vi "SetParam.vi"(8 "error in (no error)":errorcluster caption="entrée d'erreur (pas d'erreur)", 10 "zero_one_loss":cluster{"normalize":bool, "sample_weight":dbl[]}={"normalize"=TRUE, "sample_weight"=[]}, 11 "Zero_One_Loss.lvclass":refnum<class "Zero_One_Loss.lvclass">) -> (0 "error out":errorcluster caption="sortie d'erreur", 3 "Zero_One_Loss.lvclass":refnum<class "Zero_One_Loss.lvclass">)   [LabVIEW 2020, in "Zero_One_Loss.lvclass"]
doc: "Set Parameters"
uses:
  Zero_One_Loss.lvclass
  Zero_One_Loss.lvclass/Zero_One_Loss.ctl
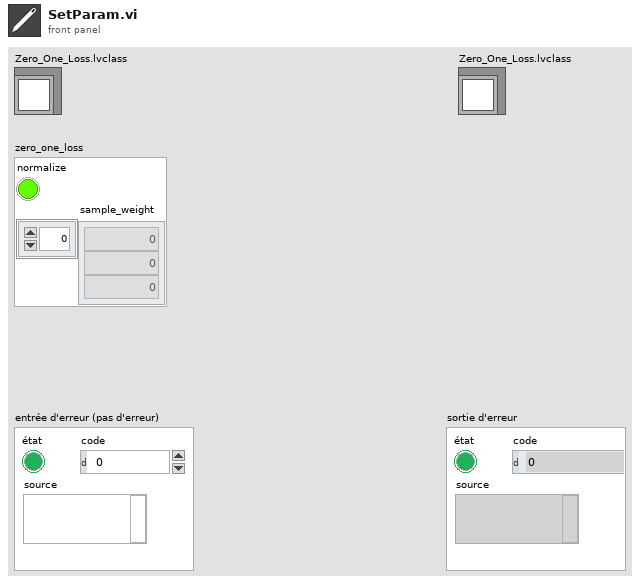
[diagram p1: front panel]
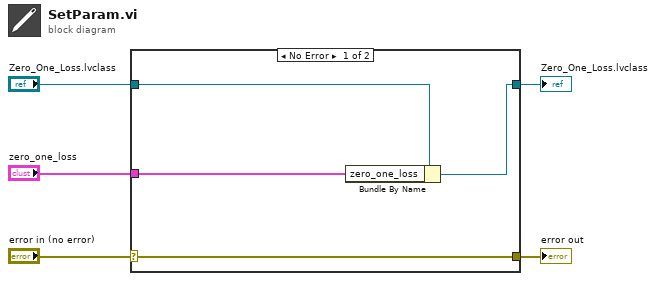
[diagram p0: block diagram]
diagram:
  n1 = case shown="No Error" "error in (no error)" {
    selector: "error in (no error)" -> [w9 w10]
    tunnel: [w9 w10] -> w4
    tunnel: [w7 w11] -> w2
    tunnel: "Zero_One_Loss.lvclass" -> [w8 w11]
    tunnel: "zero_one_loss" -> [w6 _]
    frame No Error {
      n2 = Bundle By Name(cluster=w8, "zero_one_loss"=w6) -> (w7:refnum<class "Zero_One_Loss.lvclass">)
    }
    frame Error {
    }
  }
  "error out" <- w4
  "Zero_One_Loss.lvclass" <- w2
